vi "CAN_MotorControlBMS.vi"(8 "error in (no error)":errorcluster) -> (0 "error out":errorcluster={"status"=TRUE, "code"=-61201, "source"="niLvFpga_Open_cRIO-9063.vi:6100001"})   [LabVIEW 2018]
uses:
  MotorController/Motor_Command/motorControlState.ctl
  BMS/Orion_BMS.lvclass
  MotorController/MotorController.lvclass
  BMS/Orion_BMS.lvclass/Orion_BMS.ctl
  TypeDef_LoopPeriods.ctl
  <vilib>/Platform/TimedLoop/XDataNode/timing_clust.ctl
  <vilib>/Platform/TimedLoop/XDataNode/nitl_modes.ctl
  <vilib>/Platform/TimedLoop/XDataNode/wakeup.ctl
  Control/TypeDef_DigitalOuts.ctl
  TypeDef_BMSData.ctl
  TypeDef_BMS_Status.ctl
  MotorController/MotorController.lvclass/MotorController.ctl
  MotorController/MotorData.ctl
  MotorController/MotorStatus.ctl
  <vilib>/platform/TimedLoop/XDataNode/XDataNode.xnode
  <vilib>/Platform/TimedLoop/XDataNode/XDNodeRunTimeDep.lvlib
panel:
  out "Enum":T1
  out "startDriveRes":u32
  out "stopDriveRes":u32
  out "changeTargetRes":u32
  out "targetTorqueRes":u32
  out "controlWord6Res":i16
  out "deviceFroze":bool
  out "loopCounter":i32
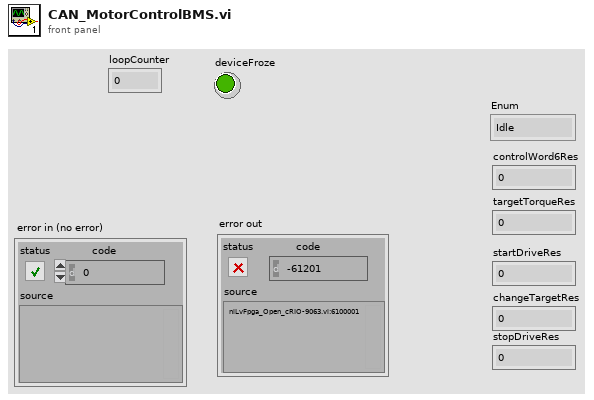
[diagram p1: front panel]
types:
  T1 = typedef "motorControlState.ctl" = enum16{"Idle", "Initialization", "Running", "Termination"}
  T2 = typedef "XDNodeRunTimeDep.lvlib/timing_clust.ctl" = cluster{"Expected End [f-1]":u64, "Actual End [f-1]":u64, "Finished Late? [f-1]":bool, "Expected End [i-1]":u64, "Actual End [i-1]":u64, "Finished Late? [i-1]":bool, "Expected Start [i]":u64, "Actual Start [i]":u64, "Expected Start [f]":u64, "Actual Start [f]":u64, "Source Name":string, "Structure Name":string, "Period":i64, "Deadline":i64, "Offset":i64, "Start":i64, "Priority":i32, "Timeout":i32, "Mode":T3, "Wakeup Reason":T4, "Error":errorcluster, "Source Type":string, "Secondary Source Type":string, "Global End Time":u64, "Global Start Time":u64, "Frame Duration":u64, "Iteration Duration":u64, "Assigned CPU":i32, "I/O Scan Engine Mode":u32}
  T3 = typedef "XDNodeRunTimeDep.lvlib/nitl_modes.ctl" = enum32{"No Change", "Process missed periods, maintain original phase", "Discard missed periods, maintain original phase", "Process missed periods, ignore original phase", "Discard missed periods, ignore original phase"}
  T4 = typedef "XDNodeRunTimeDep.lvlib/wakeup.ctl" = enum32{"Normal", "Aborted", "Asynchronous wakeup", "Timing source error", "Timed loop error", "Timeout"}
  T5 = typedef "TypeDef_LoopPeriods.ctl" = cluster{"Control Period":i64, "DAQ Period":u32, "IMU Period":u32, "CAN Period":i64, "Nav Period":u32}
  T6 = typedef "TypeDef_BMSData.ctl" = cluster{"Max Cell Voltage (V)":dbl, "Max Cell ID":dbl, "Min Cell Voltage (V)":dbl, "Min Cell ID":dbl, "State of Charge (%)":dbl, "Average Voltage (V)":dbl, "Voltage Delta (V)":dbl, "Pack Current (A)":dbl, "Pack Voltage (V)":dbl, "Max Resistance (Ohm)":dbl, "Min Resistance (Ohm)":dbl, "Average Resistance (Ohm)":dbl, "Delta Resistance (Ohm)":dbl, "Highest Temperature(F)":dbl, "BmsStatus":T7}
  T7 = typedef "TypeDef_BMS_Status.ctl" = cluster{"isFault":bool, "isolationMonitoring":bool}
  T8 = typedef "TypeDef_DigitalOuts.ctl" = cluster{"Pod Power":bool, "Dump Valve":bool, "Brakes":bool, "Clamp":bool, "Pump":bool, "Ignition":bool, "DO6":bool, "DO7":bool, "HighSide":bool, "Precharge":bool, "LowSide":bool, "DO3":bool, "DO4":bool, "DO5":bool, "DO62":bool, "DO72":bool}
  T9 = typedef "MotorData.ctl" = cluster{"Velo (RPM)":i32, "MotorTemp(C)":u8, "CtrlTemp(C)":u8, "DcLinkVolt(V)":dbl, "ErrorCode":dbl, "isAlive":bool, "motorControllerState":u16, "motorStatus":T10}
  T10 = typedef "MotorStatus.ctl" = cluster{"isReady":bool, "isOn":bool, "isOperEn":bool, "isFault":bool, "isVoltEn":bool, "targetReached":bool, "isWarning":bool}
  T11 = cluster{"error code":dbl, "error register":dbl, "manufacturer specific error field":dbl[]}
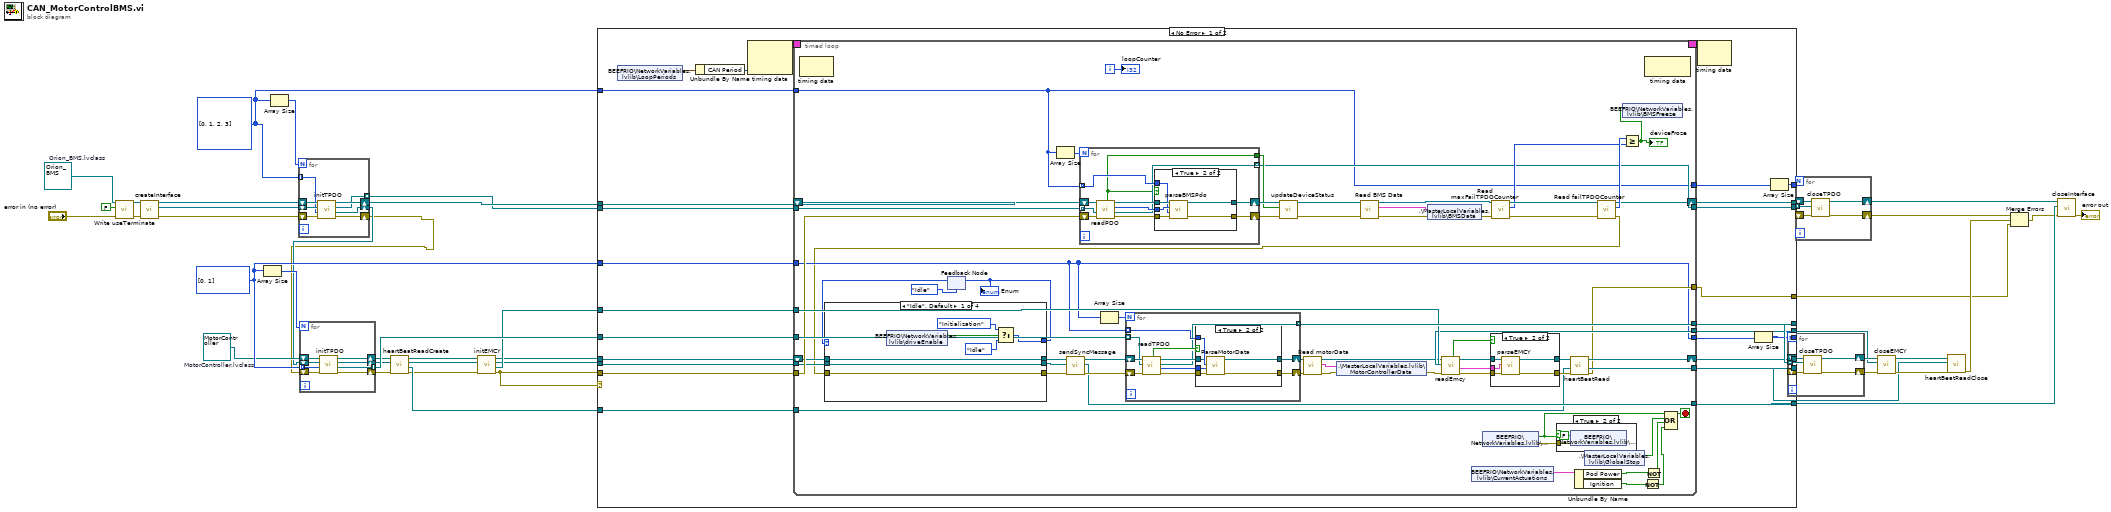
[diagram p0: block diagram]
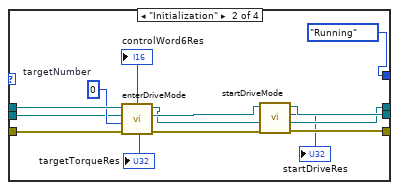
[diagram p2: hidden frame]
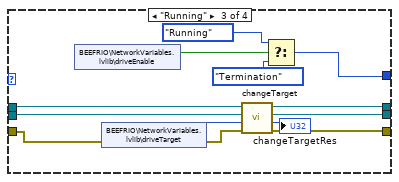
[diagram p3: hidden frame]
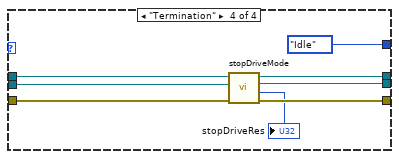
[diagram p4: hidden frame]
diagram:
  w41 = u8[] [0, 1] items=["PDO 1", "PDO 2", "PDO 3", "PDO 4"]
  w18 = refnum<class "MotorController.lvclass"> refnum  # MotorController.lvclass
  w6 = refnum<class "Orion_BMS.lvclass"> refnum  # Orion_BMS.lvclass
  w48 = u8[] [0, 1, 2, 3] items=["PDO 1", "PDO 2", "PDO 3", "PDO 4"]
  n1 = call "Write useTerminate.vi"("error in (no error)"="error in (no error)", "useTerminate"=FALSE, "Orion_BMS in"=w6) -> ("error out"=w8:errorcluster, "Orion_BMS out"=w9:refnum<class "Orion_BMS.lvclass">)  [unwired: 7 in]
  n2 = call "createInterface.vi"("error in (no error)"=w8, "Orion_BMS in"=w9) -> ("error out"=w10:errorcluster, "interface object out"=w19:refnum<k20>, "Orion_BMS out"=w20:refnum<class "Orion_BMS.lvclass">)  [unwired: 7 in]
  n3 = Array Size(array=w41) -> (size(s)=w42:i32)
  n4 = Array Size(array=w48) -> (size(s)=w43:i32)
  n5 = for {
    N: w43 -> [_]
    tunnel: w48 -> [w55] mode=indexing
    shift-right: [w52] -> w17
    shift-left: w19 -> [w56]
    tunnel: [w51] -> w49 mode=indexing
    shift-right: [w53] -> w50
    shift-left: w20 -> [w58]
    shift-right: [w54] -> w1
    shift-left: w10 -> [w57]
    n6 = call "initTPDO.vi"("error in (no error)"=w57, "PDO channel"=w55, "interface object in"=w56, "Orion_BMS in"=w58) -> ("error out"=w54:errorcluster, "interface object out"=w52:refnum<k20>, "TPDO object out"=w51:refnum<k20>, "Orion_BMS out"=w53:refnum<class "Orion_BMS.lvclass">)  [unwired: 4 in]
  }
  n7 = for {
    N: w42 -> [_]
    tunnel: w41 -> [w64] mode=indexing
    shift-right: [w62] -> w13
    shift-left: w17 -> [w63]
    tunnel: [w61] -> w40 mode=indexing
    shift-right: [w59] -> w11
    shift-left: w1 -> [w60]
    shift-right: [w65] -> w12
    shift-left: w18 -> [w66]
    n8 = call "initTPDO.vi"("error in (no error)"=w60, "PDO channel"=w64, "interface object in"=w63, "MotorController in"=w66) -> ("error out"=w59:errorcluster, "TPDO object out"=w61:refnum<k20>, "interface object out"=w62:refnum<k20>, "MotorController out"=w65:refnum<class "MotorController.lvclass">)  [unwired: 4 in]
  }
  n9 = call "heartBeatReadCreate.vi"("error in (no error)"=w11, "interface object in"=w13, "MotorController in"=w12) -> ("error out"=w15:errorcluster, "heartbeat object out"=w37:refnum<k20>, "interface object out"=w16:refnum<k20>, "MotorController out"=w14:refnum<class "MotorController.lvclass">)  [unwired: 5 in]
  n10 = call "initEMCY.vi"("error in (no error)"=w15, "interface object in"=w16, "MotorController in"=w14) -> ("error out"=w2:errorcluster, "emergency object out"=w38:refnum<k20>, "interface object out"=w4:refnum<k20>, "MotorController out"=w3:refnum<class "MotorController.lvclass">)  [unwired: 5 in]
  n11 = case shown="No Error" w2 {
    tunnel: w50 -> [w86 w259]
    tunnel: w49 -> [w85 w258]
    tunnel: w48 -> [w84 w260]
    tunnel: [w83 w260] -> w46
    tunnel: [w82 w259] -> w45
    tunnel: [w81 w258] -> w44
    tunnel: w41 -> [w80 w257]
    tunnel: w40 -> [w79 w253]
    tunnel: [w68 w251] -> w39
    tunnel: w4 -> [w70 w251]
    tunnel: w3 -> [w71 w256]
    tunnel: w38 -> [w78 w252]
    tunnel: w37 -> [w77 w254]
    tunnel: [w69 w256] -> w32
    tunnel: [w76 w252] -> w30
    tunnel: [w75 w254] -> w29
    tunnel: [w74 w253] -> w27
    tunnel: w2 -> [w72 w255]
    tunnel: [w67 w255] -> w23
    tunnel: [w73 w257] -> w21
    frame No Error {
      n12 = shared-variable "BEEFRIO\\NetworkVariables.lvlib\\LoopPeriods"() -> (w88:T5)  [unwired: 1 in, 1 out]
      n13 = Unbundle By Name(w88) -> ("CAN Period"=w87:i64)
      n14 = node-c288(w87) -> (w90:T2)  [unwired: 1 in]
      n15 = timed-loop {
        timing: w90 -> [_]
        timing-out: [_] -> w89
        tunnel: w85 -> [w154]
        tunnel: w84 -> [w105]
        tunnel: [w139] -> w81
        tunnel: [w105] -> w83
        tunnel: w80 -> [w103]
        tunnel: w79 -> [w138]
        tunnel: [w137] -> w74
        tunnel: w70 -> [w96]
        tunnel: [w134] -> w68
        tunnel: w78 -> [w129]
        tunnel: w77 -> [w126]
        tunnel: [w124] -> w76
        tunnel: [w123] -> w75
        tunnel: w72 -> [w118]
        tunnel: [w103] -> w73
        tunnel: [w116] -> w67
        shift-right: [w125] -> w69
        shift-left: w71 -> [w97]
        shift-right: [w140] -> w82
        shift-left: w86 -> [w155]
        i -> [w119]
        stop <- w117 stop-if-true
        n16 = node-c288() -> ()  [unwired: 1 in, 1 out]
        n17 = feedback #1(motorControlState."Idle") -> (w99:T1)
        n18 = Array Size(array=w105) -> (size(s)=w106:i32)
        n19 = for {
          N: w106 -> [_]
          shift-right: [w228] -> w153
          shift-left: w118 -> [w233]
          tunnel: w154 -> [w231] mode=indexing
          tunnel: w105 -> [w230] mode=indexing
          shift-right: [w229] -> w152
          shift-left: w155 -> [w232]
          tunnel: [w226] -> w151
          tunnel: [w227] -> w139 mode=indexing
          n20 = call "readPDO.vi"("error in (no error)"=w233, "TPDO object in"=w231, "Orion_BMS in"=w232) -> ("error out"=w236:errorcluster, "TPDO object out"=w227:refnum<k20>, "TPDO data"=w235:u8[], "Orion_BMS out"=w234:refnum<class "Orion_BMS.lvclass">, "new data?"=w226:bool)  [unwired: 4 in]
          n21 = case shown="True" w226 {
            tunnel: w236 -> [w237 w244]
            tunnel: w235 -> [_ w243]
            tunnel: w234 -> [w238 w242]
            tunnel: w230 -> [_ w241]
            tunnel: [w238 w240] -> w229
            tunnel: [w237 w239] -> w228
            frame False {
            }
            frame True {
              n22 = call "parseBMSPdo.vi"("error in (no error)"=w244, "PDO channel"=w241, "TPDO data"=w243, "Orion_BMS in"=w242) -> ("error out"=w239:errorcluster, "Orion_BMS out"=w240:refnum<class "Orion_BMS.lvclass">)  [unwired: 6 in]
            }
          }
        }
        n23 = Array Size(array=w103) -> (size(s)=w104:i32)
        n24 = call "updateDeviceStatus.vi"("error in (no error)"=w153, "isNewData"=w151, "Orion_BMS in"=w152) -> ("error out"=w143:errorcluster, "Orion_BMS out"=w142:refnum<class "Orion_BMS.lvclass">)  [unwired: 7 in]
        n25 = call "Read BMS Data.vi"("error in (no error)"=w143, "Orion_BMS in"=w142) -> ("error out"=w149:errorcluster, "BMS Data"=w148:T6, "Orion_BMS out"=w144:refnum<class "Orion_BMS.lvclass">)  [unwired: 7 in]
        n26 = shared-variable ".\\MasterLocalVariables.lvlib\\BMSData"(w148, error in=w149) -> (error out=w150:errorcluster)
        n27 = shared-variable "BEEFRIO\\NetworkVariables.lvlib\\CurrentActuations"() -> (w115:T8)  [unwired: 1 in, 1 out]
        n28 = shared-variable "BEEFRIO\\NetworkVariables.lvlib\\ReintCAN"() -> (w107:bool, error out=w108:errorcluster)  [unwired: 1 in]
        n29 = call "Read maxFailTPDOCounter.vi"("error in (no error)"=w150, "Orion_BMS in"=w144) -> ("error out"=w146:errorcluster, "maxFailTPDOCounter"=w141:u8, "Orion_BMS out"=w145:refnum<class "Orion_BMS.lvclass">)  [unwired: 7 in]
        n30 = case shown="True" w107 {
          tunnel: w108 -> [_ w199]
          frame False {
          }
          frame True {
            n31 = shared-variable "BEEFRIO\\NetworkVariables.lvlib\\ReintCAN"(FALSE ("ReintCAN"), error in=w199) -> ()  [unwired: 1 out]
          }
        }
        n32 = Unbundle By Name(w115) -> ("Pod Power"=w114:bool, "Ignition"=w102:bool)
        n33 = shared-variable ".\\MasterLocalVariables.lvlib\\GlobalStop"() -> (w109:bool)  [unwired: 1 in, 1 out]
        n34 = call "Read failTPDOCounter.vi"("error in (no error)"=w146, "Orion_BMS in"=w145) -> ("error out"=w92:errorcluster, "failTPDOCounter"=w147:u32, "Orion_BMS out"=w140:refnum<class "Orion_BMS.lvclass">)  [unwired: 7 in]
        n35 = case shown="\"Idle\", Default" w99 {
          tunnel: w97 -> [w158 w176 w185 w191]
          tunnel: [w158 w167 w184 w196] -> w93
          tunnel: [w157 w164 w181 w194] -> w95
          tunnel: w92 -> [w157 w175 w179 w193]
          tunnel: [w156 w168 w183 w195] -> w94
          tunnel: w96 -> [w156 w173 w182 w192]
          tunnel: [w161 motorControlState."Running" w187 motorControlState."Idle"] -> w98
          frame "Idle", Default {
            n36 = shared-variable "BEEFRIO\\NetworkVariables.lvlib\\driveEnable"() -> (w162:bool)  [unwired: 1 in, 1 out]
            n37 = Select(t=motorControlState."Initialization", s=w162, f=motorControlState."Idle") -> (s? t:f=w161:T1)
          }
          frame "Initialization" {
            w174 = i16 0  # targetNumber
            n38 = call "enterDriveMode.vi"("error in (no error)"=w175, "targetNumber"=w174, "interface object in"=w173, "MotorController in"=w176) -> ("error out"=w165:errorcluster, "interface object out"=w169:refnum<k20>, "MotorController out"=w166:refnum<class "MotorController.lvclass">, "targetTorqueRes"=→"targetTorqueRes":u32, "controlWord6Res"=→"controlWord6Res":i16)  [unwired: 3 in]
            n39 = call "startDriveMode.vi"("error in (no error)"=w165, "MotorController in"=w166, "interface object in"=w169) -> ("error out"=w164:errorcluster, "MotorController out"=w167:refnum<class "MotorController.lvclass">, "startDriveRes"=→"startDriveRes":u32, "interface object out"=w168:refnum<k20>)  [unwired: 5 in]
          }
          frame "Running" {
            n40 = shared-variable "BEEFRIO\\NetworkVariables.lvlib\\driveEnable"() -> (w186:bool)  [unwired: 1 in, 1 out]
            n41 = shared-variable "BEEFRIO\\NetworkVariables.lvlib\\driveTarget"(error in=w179) -> (w180:i16, error out=w178:errorcluster)
            n42 = call "changeTarget.vi"("error in (no error)"=w178, "targetNumber"=w180, "interface object in"=w182, "MotorController in"=w185) -> ("error out"=w181:errorcluster, "changeTargetRes"=→"changeTargetRes":u32, "interface object out"=w183:refnum<k20>, "MotorController out"=w184:refnum<class "MotorController.lvclass">)  [unwired: 4 in]
            n43 = Select(t=motorControlState."Running", s=w186, f=motorControlState."Termination") -> (s? t:f=w187:T1)
          }
          frame "Termination" {
            n44 = call "stopDriveMode.vi"("error in (no error)"=w193, "interface object in"=w192, "MotorController in"=w191) -> ("error out"=w194:errorcluster, "stopDriveRes"=→"stopDriveRes":u32, "interface object out"=w195:refnum<k20>, "MotorController out"=w196:refnum<class "MotorController.lvclass">)  [unwired: 5 in]
          }
        }
        "Enum" <- w98
        n45 = feedback-in #1(w98) -> ()
        n46 = call "sendSyncMessage.vi"("error in (no error)"=w95, "interface object in"=w94, "MotorController in"=w93) -> ("error out"=w136:errorcluster, "interface object out"=w134:refnum<k20>, "MotorController out"=w135:refnum<class "MotorController.lvclass">)  [unwired: 6 in]
        n47 = for {
          N: w104 -> [_]
          tunnel: w103 -> [w216] mode=indexing
          shift-right: [w213] -> w122
          shift-left: w135 -> [w217]
          shift-right: [w211] -> w121
          shift-left: w136 -> [w212]
          tunnel: w138 -> [w208] mode=indexing
          tunnel: [w207] -> w137 mode=indexing
          n48 = call "readTPDO.vi"("error in (no error)"=w212, "TPDO object in"=w208, "MotorController in"=w217) -> ("error out"=w215:errorcluster, "TPDO data"=w210:u8[], "TPDO object out"=w207:refnum<k20>, "MotorController out"=w214:refnum<class "MotorController.lvclass">, "new data?"=w209:bool)  [unwired: 4 in]
          n49 = case shown="True" w209 {
            tunnel: w216 -> [_ w225]
            tunnel: w215 -> [w218 w224]
            tunnel: w214 -> [w219 w223]
            tunnel: [w219 w222] -> w213
            tunnel: [w218 w221] -> w211
            tunnel: w210 -> [_ w220]
            frame False {
            }
            frame True {
              n50 = call "ParseMotorData.vi"("error in (no error)"=w224, "TPDO data"=w220, "PDO channel"=w225, "MotorController in"=w223) -> ("error out"=w221:errorcluster, "MotorController out"=w222:refnum<class "MotorController.lvclass">)  [unwired: 6 in]
            }
          }
        }
        n51 = call "Read motorData.vi"("error in (no error)"=w121, "MotorController in"=w122) -> ("error out"=w112:errorcluster, "motorData"=w111:T9, "MotorController out"=w120:refnum<class "MotorController.lvclass">)  [unwired: 7 in]
        n52 = shared-variable ".\\MasterLocalVariables.lvlib\\MotorControllerData"(w111, error in=w112) -> (error out=w110:errorcluster)
        n53 = call "readEmcy.vi"("error in (no error)"=w110, "emergency object in"=w129, "MotorController in"=w120) -> ("error out"=w133:errorcluster, "emergency message"=w131:T11, "emergency object out"=w124:refnum<k20>, "MotorController out"=w132:refnum<class "MotorController.lvclass">, "isNewMessage"=w130:bool)  [unwired: 4 in]
        n54 = case shown="True" w130 {
          tunnel: w132 -> [w201 w206]
          tunnel: w133 -> [w200 w205]
          tunnel: w131 -> [_ w204]
          tunnel: [w201 w203] -> w128
          tunnel: [w200 w202] -> w127
          frame False {
          }
          frame True {
            n55 = call "parseEMCY.vi"("error in (no error)"=w205, "emergency message"=w204, "MotorController in"=w206) -> ("error out"=w202:errorcluster, "MotorController out"=w203:refnum<class "MotorController.lvclass">)  [unwired: 7 in]
          }
        }
        n56 = call "heartBeatRead.vi"("error in (no error)"=w127, "heartbeat object in"=w126, "MotorController in"=w128) -> ("error out"=w116:errorcluster, "heartbeat object out"=w123:refnum<k20>, "MotorController out"=w125:refnum<class "MotorController.lvclass">)  [unwired: 6 in]
        n57 = Greater Or Equal?(x=w147, y=w141) -> (x >= y?=w91:bool)
        "deviceFroze" <- w91
        n58 = shared-variable "BEEFRIO\\NetworkVariables.lvlib\\BMSFreeze"(w91) -> ()  [unwired: 1 in, 1 out]
        n59 = Not(x=w102) -> (.not. x?=w101:bool)
        n60 = node-c288() -> ()  [unwired: 1 in, 1 out]
        n61 = Not(x=w114) -> (.not. x?=w113:bool)
        n62 = Compound Arithmetic op=OR(w107, w109, w113, w101) -> (w117:bool)
        "loopCounter" <- w119
      }
      n63 = node-c288(w89) -> ()  [unwired: 1 out]
    }
    frame Error {
    }
  }
  n64 = Array Size(array=w21) -> (size(s)=w22:i32)
  n65 = Array Size(array=w46) -> (size(s)=w47:i32)
  n66 = for {
    N: w22 -> [_]
    shift-right: [w264] -> w33
    shift-left: _ -> [w265]
    shift-right: [w262] -> w31
    shift-left: w32 -> [w263]
    tunnel: w27 -> [w261] mode=indexing
    n67 = call "closeTPDO.vi"("error in (no error)"=w265, "TPDO object in"=w261, "MotorController in"=w263) -> ("error out"=w264:errorcluster, "MotorController out"=w262:refnum<class "MotorController.lvclass">)  [unwired: 7 in]
  }
  n68 = for {
    N: w47 -> [_]
    shift-right: [w266] -> w26
    shift-left: _ -> [w270]
    shift-right: [w268] -> w36
    shift-left: w45 -> [w269]
    tunnel: w44 -> [w267] mode=indexing
    n69 = call "closeTPDO.vi"("error in (no error)"=w270, "TPDO object in"=w267, "Orion_BMS in"=w269) -> ("error out"=w266:errorcluster, "Orion_BMS out"=w268:refnum<class "Orion_BMS.lvclass">)  [unwired: 7 in]
  }
  n70 = call "closeEMCY.vi"("error in (no error)"=w33, "emergency object in"=w30, "MotorController in"=w31) -> ("error out"=w34:errorcluster, "MotorController out"=w35:refnum<class "MotorController.lvclass">)  [unwired: 7 in]
  n71 = call "heartBeatReadClose.vi"("error in (no error)"=w34, "heartbeat object in"=w29, "MotorController in"=w35) -> ("error out"=w25:errorcluster)  [unwired: 7 in, 1 out]
  n72 = Merge Errors(w26, w25, w23) -> (w24:errorcluster)
  n73 = call "closeInterface.vi"("error in (no error)"=w24, "interface object in"=w39, "Orion_BMS in"=w36) -> ("error out"=→"error out":errorcluster)  [unwired: 7 in, 1 out]
